vi "AMZ_S3_APIHLP_Generate Filter Rule XML.vi"(11 "Filter Rules":T1[](array[typedef])) -> (3 "Filter Rule XML":string)   [LabVIEW 2015, in "LV Interface for Amazon S3.lvlib"]
uses:
  LV Interface for Amazon S3.lvlib
  Typedefs/AMZ_S3_FilterRule.ctl
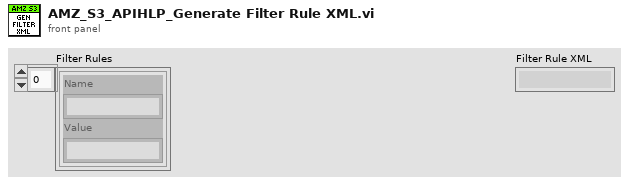
[diagram p1: front panel]
types:
  T1 = typedef "LV Interface for Amazon S3.lvlib/AMZ_S3_FilterRule.ctl" = cluster{"Name":string, "Value":string}
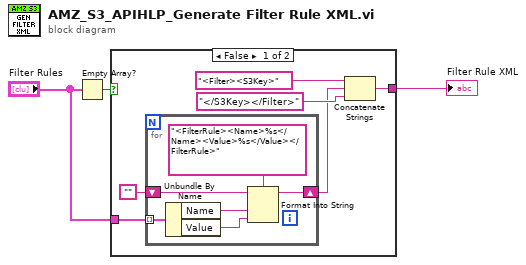
[diagram p0: block diagram]
diagram:
  n1 = Empty Array?(array="Filter Rules") -> (empty?=w1:bool)
  n2 = case shown="False" w1 {
    tunnel: "Filter Rules" -> [w6 _]
    tunnel: [w7 _] -> w3
    frame False {
      n3 = for {
        tunnel: w6 -> [w15] mode=indexing
        shift-right: [w13] -> w4
        shift-left: "" -> [w14]
        n4 = Unbundle By Name(w15) -> ("Name"=w12:string, "Value"=w11:string)
        n5 = Format Into String(format string="<FilterRule><Name>%s</Name><Value>%s</Value></FilterRule>", initial string=w14, w12, w11) -> (resulting string=w13:string)  [unwired: 1 in, 1 out]
      }
      n6 = Concatenate Strings("<Filter><S3Key>", w4, "</S3Key></Filter>") -> (w7:string)
    }
    frame True {
    }
  }
  "Filter Rule XML" <- w3
